vi "Toggle Selection Of An Object.vi"   [LabVIEW 2023]
doc: "Demonstrates the use of the Selected property in VI Scripting to read and write the selection status of an individual object."
uses:
  <vilib>/Utility/traverseref.llb/TRef TravTarget.ctl
  <vilib>/Utility/traverseref.llb/VI Scripting - Traverse.lvlib
panel:
  # "Overview: Demonstrates the use of the Selected property in VI Scripting to read and write the selection status of an individual object.\nInstructions:\n1. Open the front panel of Test - Selection List Target.vi.\n2. Select one or more objects.\n3. Run this VI. The objects you selected will become deselected, and the objects you did not select will become selected. To see this, click the front panel window title bar of the Test - Selection List Target.vi after running this VI to make it the active window."
types:
  T1 = typedef "TRef TravTarget.ctl" = enum16{"FP", "BD", "Other"}
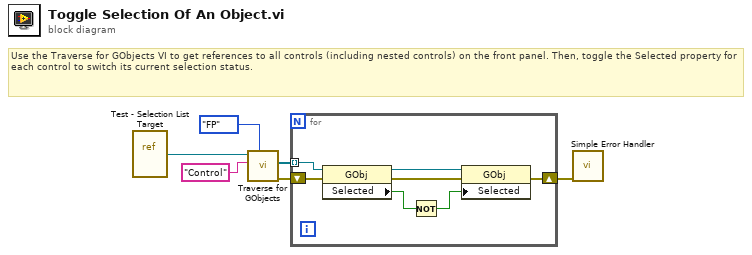
[diagram p0: block diagram]
diagram:
  # "Use the Traverse for GObjects VI to get references to all controls (including nested controls) on the front panel. Then, toggle the Selected property for each control to switch its current selection status."
  n1 = vi-ref "Test - Selection List Target.vi"() -> (w6:refnum<vi>)
  n2 = call <vilib>:"Traverse for GObjects.vi"("Traverse Target"=TRef_TravTarget."FP", "Class Name"="Control", "VI Refnum"=w6) -> ("error out"=w3:errorcluster, "References"=w2:refnum<vi>[])  [unwired: 5 in, 2 out]
  n3 = for {
    shift-right: [w7] -> w1
    shift-left: w3 -> [w11]
    tunnel: w2 -> [w10] mode=indexing
    n4 = property class="GObj"(reference=w10, error in=w11) -> (reference out=w13:refnum<vi>, error out=w9:errorcluster, "Selected"=w8:bool)
    n5 = Not(x=w8) -> (.not. x?=w12:bool)
    n6 = property class="GObj"(reference=w13, error in=w9, "Selected"=w12) -> (error out=w7:errorcluster)  [unwired: 1 out]
  }
  n7 = call <vilib>:"Simple Error Handler.vi"("error in (no error)"=w1) -> ()  [unwired: 4 in, 5 out]
